vi "XYZStage.vi"() -> ()   [LabVIEW 2016]
uses:
  controls/Enum.ctl
  <vilib>/rvi/errors/niLvFpgaAdjustHostInterfaceError.vi
  <vilib>/rvi/interface/nirviReadWriteControl/nirviReadWriteControl.xnode
  controls/FPGAVIreferenceTypeDefScanEngine.ctl
  FPGA Bitfiles/lbniAFMControlle_scanControl_controllerFPGAPX_N4i+37z1gG8.lvbitx
  Course Project/support/Message Queue/Message Queue.lvlib
  NiFpgaLv.dll
panel:
  in  "x N (Discrete)":i32
  in  "Z axis":cluster{"Amplitude":dbl, "Frequency (Hz)":dbl}={"Amplitude"=0.1, "Frequency (Hz)"=100.0} {"Frequency (Hz)" scale=1.0..5000.0; "Amplitude" scale=0.0..10.0}
  in  "Z":cluster{"+":bool, "-":bool}
  in  "ClockDivider":i16=40
  in  "Increment":i16=30
  in  "Target":i16=30
  out "Output Scale":fxp<+/-,16,16>=16390.0
  in  "Max x":i16=32767
  in  "Min x":i16=-32767
  in  "Steps in a ramp":i16=31380
  in  "Steps":i16=32767
  in  "Y axis":cluster{"Amplitude":dbl, "Frequency (Hz)":dbl}={"Amplitude"=0.1, "Frequency (Hz)"=100.0} {"Frequency (Hz)" scale=1.0..5000.0; "Amplitude" scale=0.0..10.0}
  in  "X axis":cluster{"Amplitude":dbl, "Frequency (Hz)":dbl}={"Amplitude"=0.1, "Frequency (Hz)"=100.0} {"Frequency (Hz)" scale=1.0..5000.0; "Amplitude" scale=0.0..10.0}
  in  "X":cluster{"+":bool, "-":bool, "Stop":bool}
  in  "Y":cluster{"+":bool, "-":bool}
  in  "lock XY":bool
  in  "continuous":bool
  # "Joystick"
  # "XY stage"
  # "Z stage"
  # "Continuous"
  # "Discrete"
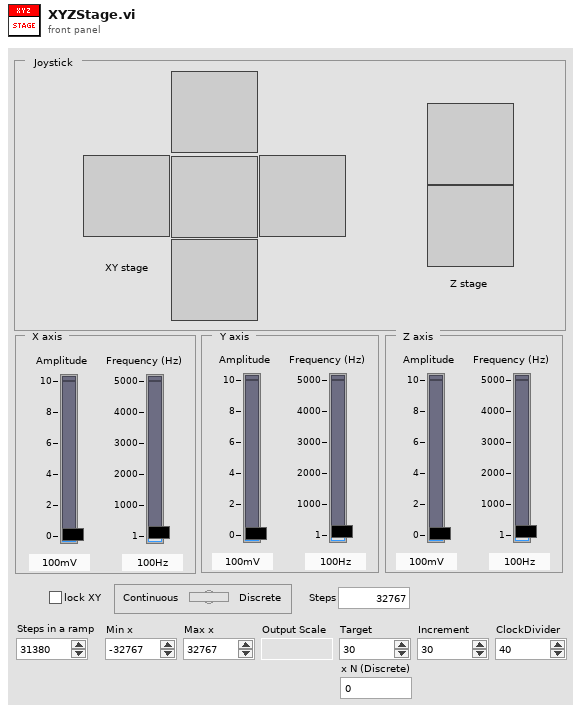
[diagram p1: front panel]
types:
  T1 = typedef "Message Queue.lvlib/All Message Queues.ctl" = cluster{"IU":refnum<queue>}
  T2 = typedef "Enum.ctl" = enum16{"Init", "Read", "Write"}
  T3 = typedef "FPGAVIreferenceTypeDefScanEngine.ctl" = refnum<k20>
  T4 = cluster{"InitialX":fxp<+/-,16,16>, "InitialY":fxp<+/-,16,16>, "InitialZ":fxp<+/-,16,16>}
  T5 = cluster{"target ":i16, "increment":i16, "ClockDivider":i16, "axis":enum16{"none", "x", "y", "z"}}
  T6 = cluster{"min_x":i16, "max_x":i16, "Total number of ramps":i16, "OutputScale":fxp<+/-,16,16>, "Steps in a ramp":i16}
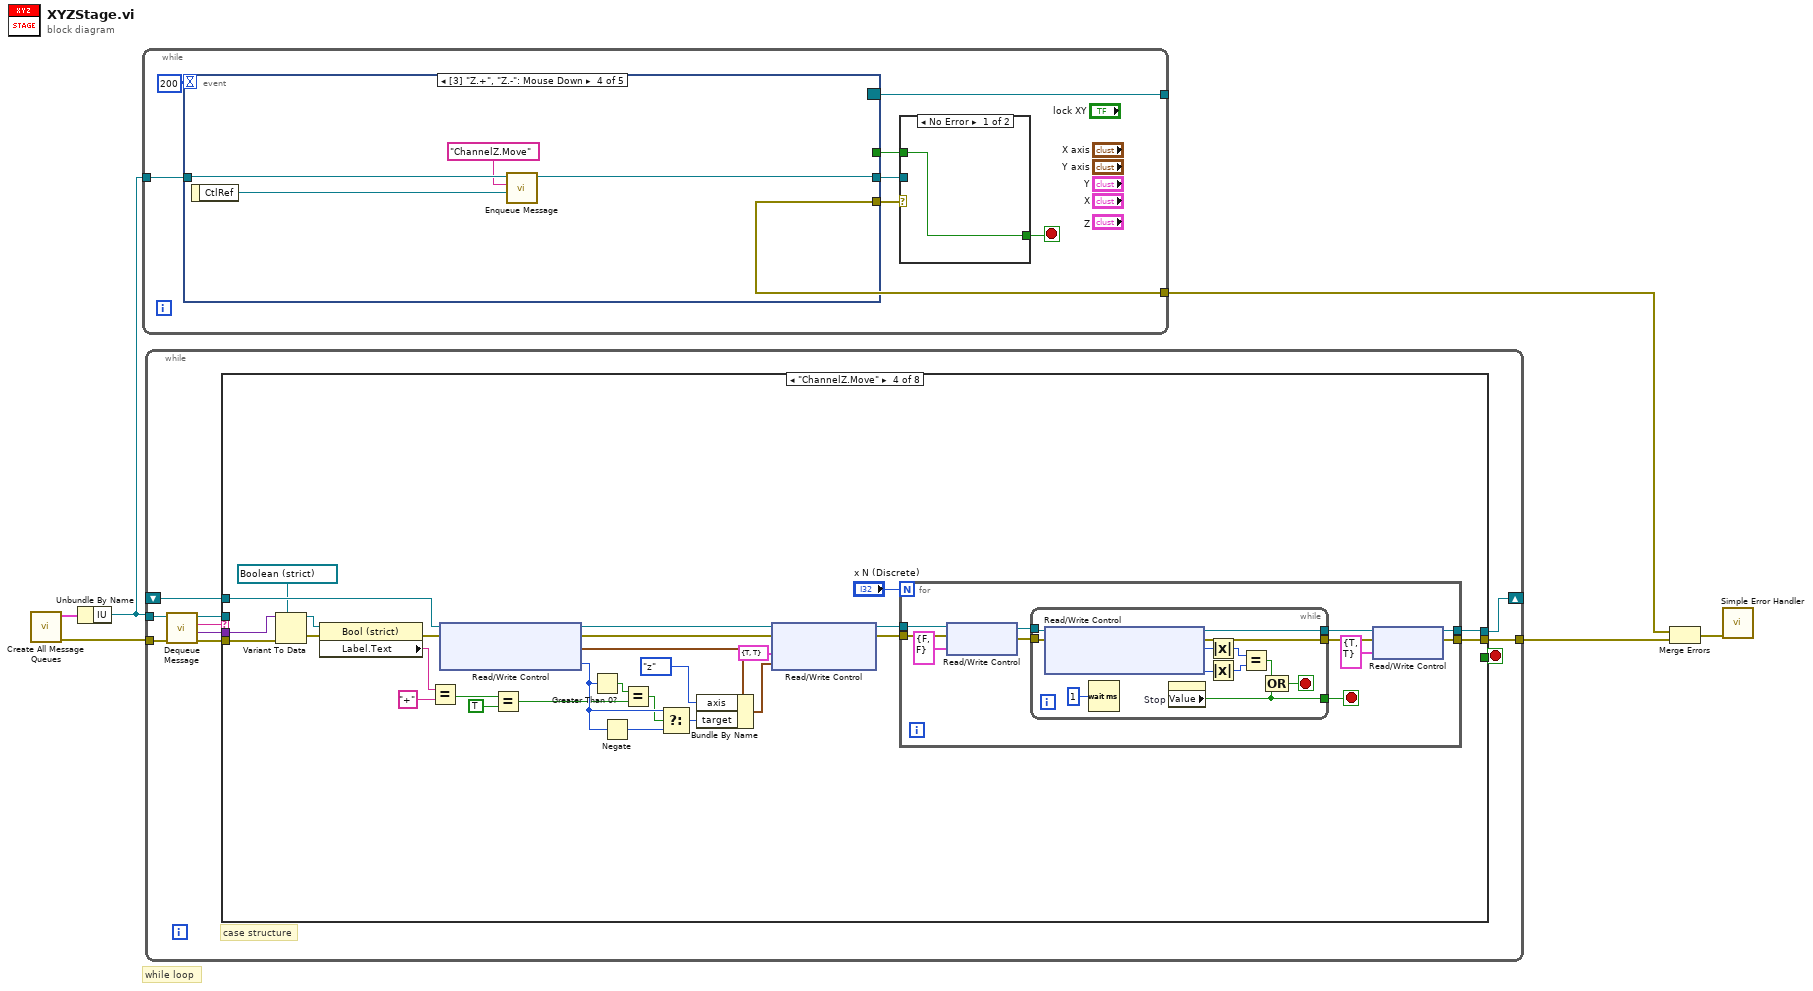
[diagram p0: block diagram]
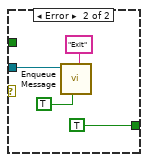
[diagram p2: hidden frame]
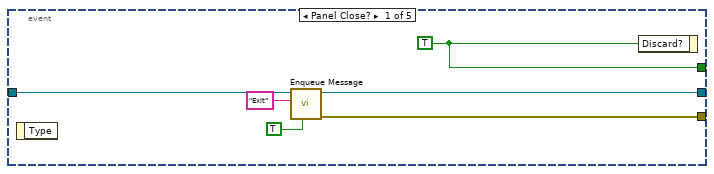
[diagram p3: hidden frame]
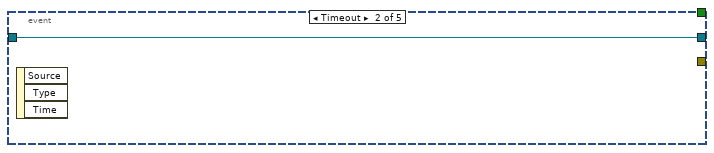
[diagram p4: hidden frame]
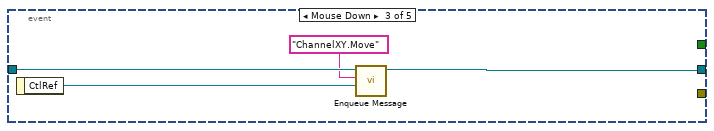
[diagram p5: hidden frame]
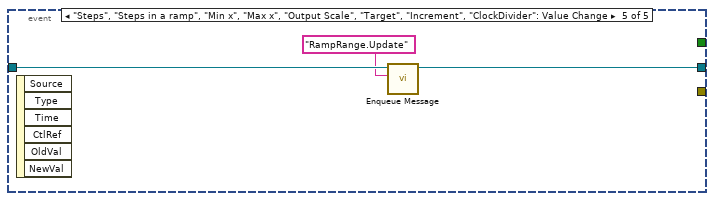
[diagram p6: hidden frame]
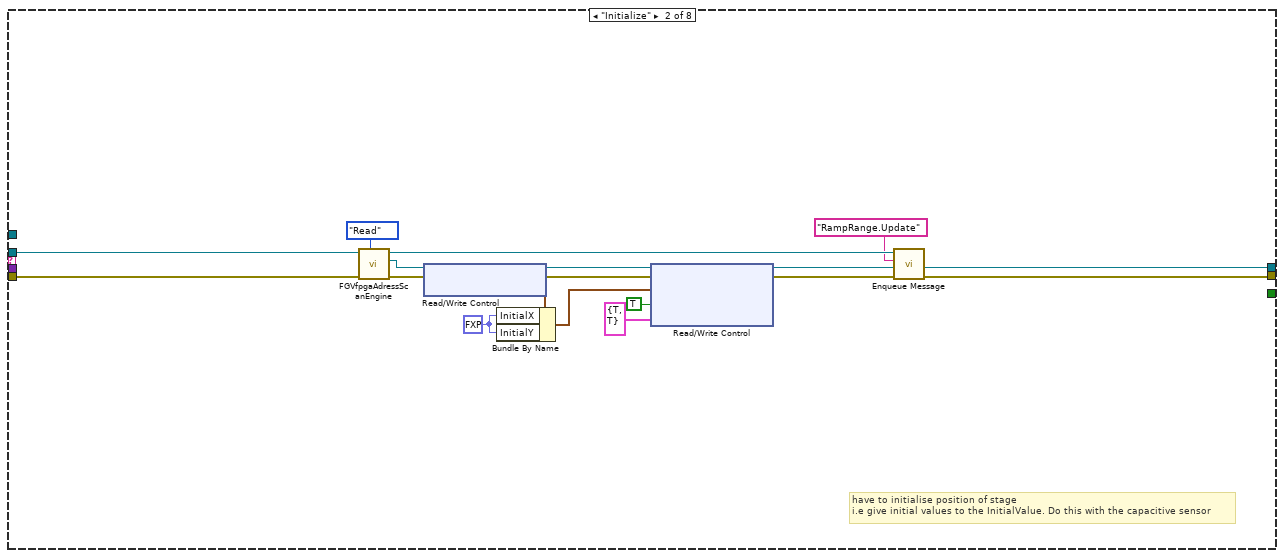
[diagram p8: hidden frame]
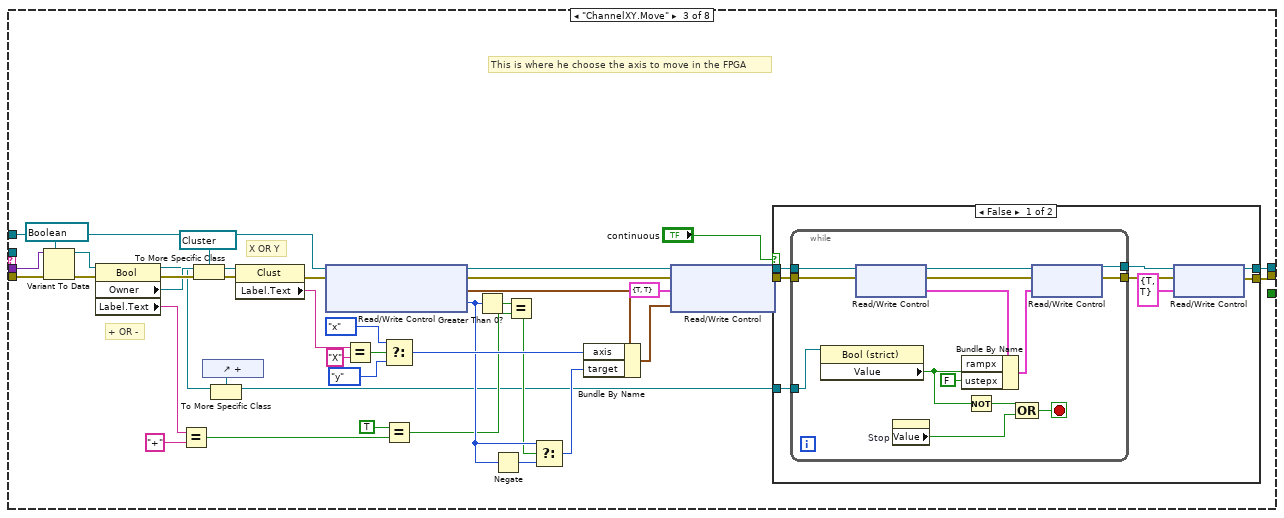
[diagram p9: hidden frame]
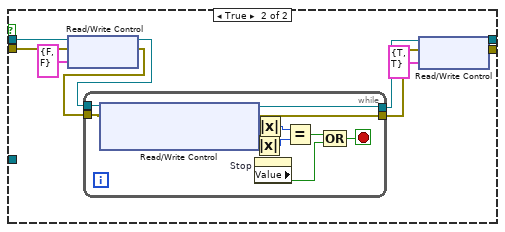
[diagram p10: hidden frame]
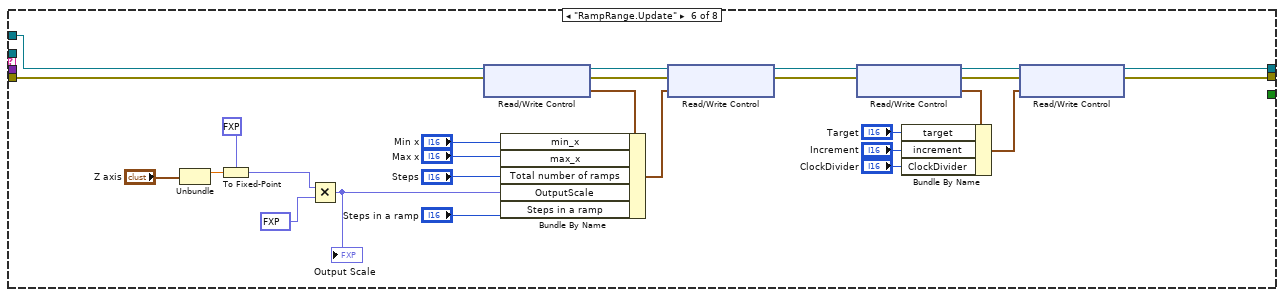
[diagram p12: hidden frame]
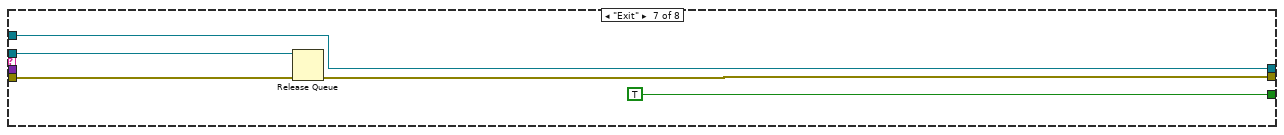
[diagram p13: hidden frame]
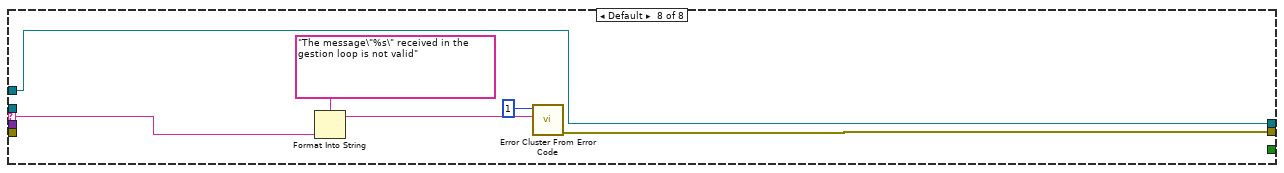
[diagram p14: hidden frame]
diagram:
  # "while loop"
  n1 = call "Create All Message Queues.vi"() -> ("ErrorOut"=w4:errorcluster, "MessageQueueOut"=w6:T1)  [unwired: 10 in]
  n2 = Unbundle By Name(w6) -> ("IU"=w5:refnum<queue>)
  n3 = while {
    tunnel: w5 -> [w13]
    tunnel: [w9] -> w1
    tunnel: [w8] -> _
    stop <- w11 stop-if-true
    n4 = event shown="[3] \"Z.+\", \"Z.-\": Mouse Down" {
      selector: _ -> [_ _ _ _ _]
      dyn-events: [_ _ _ _ _] -> w8
      timeout: 200 -> [_ _ _ _ _]
      tunnel: [w24 _ _ _ _] -> w12
      tunnel: w13 -> [w23 w25 w29 w33 w36]
      tunnel: [w22 _ _ _ _] -> w9
      tunnel: [w21 w25 w26 w31 w35] -> w10
      event Panel Close? {
        w24 = TRUE ("Rejeter ?")
        n5 = event-data() -> ()  [unwired: 1 in, 1 out]
        n6 = call "Enqueue Message.vi"("Prioritary message"=TRUE ("Message prioritaire ? (F)"), "Message"="Exit", "Queue"=w23) -> ("error out"=w22:errorcluster, "Queue dup."=w21:refnum<queue>)  [unwired: 7 in]
        n7 = event-data ("Event Filter Node")("Discard?"=w24) -> ()  [unwired: 1 in, 1 out]
      }
      event Timeout {
        n8 = event-data() -> ()  [unwired: 1 in, 3 out]
      }
      event "Y.+", "Y.-", "X.+", "X.-": Mouse Down {
        n9 = event-data() -> ("CtlRef"=w28:refnum<vi>)  [unwired: 1 in]
        n10 = call "Enqueue Message.vi"("Data"=w28, "Message"="ChannelXY.Move", "Queue"=w29) -> ("Queue dup."=w26:refnum<queue>)  [unwired: 7 in, 1 out]
      }
      event "Z.+", "Z.-": Mouse Down {
        n11 = event-data() -> ("CtlRef"=w30:refnum<vi>)  [unwired: 1 in]
        n12 = call "Enqueue Message.vi"("Data"=w30, "Message"="ChannelZ.Move", "Queue"=w33) -> ("Queue dup."=w31:refnum<queue>)  [unwired: 7 in, 1 out]
      }
      event "Steps", "Steps in a ramp", "Min x", "Max x", "Output Scale", "Target", "Increment", "ClockDivider", "Z axis.Amplitude": Value Change {
        n13 = event-data() -> ()  [unwired: 1 in, 6 out]
        n14 = call "Enqueue Message.vi"("Message"="RampRange.Update", "Queue"=w36) -> ("Queue dup."=w35:refnum<queue>)  [unwired: 8 in, 1 out]
      }
    }
    n15 = case shown="No Error" w9 {
      tunnel: [w14 TRUE ("Rejeter ?")] -> w11
      tunnel: w12 -> [w14 _]
      tunnel: w10 -> [_ w17]
      frame No Error {
      }
      frame Error {
        n16 = call "Enqueue Message.vi"("Prioritary message"=TRUE ("Message prioritaire ? (F)"), "Message"="Exit", "Queue"=w17) -> ()  [unwired: 7 in, 2 out]
      }
    }
  }
  n17 = while {
    tunnel: w5 -> [w40]
    tunnel: w4 -> [w44]
    tunnel: [w45] -> w2
    shift-right: [w38] -> _
    shift-left: _ -> [w37]
    stop <- w46 stop-if-true
    # "case structure"
    n18 = call "Dequeue Message.vi"("entrée d'erreur (pas d'erreur)"=w44, "File d'attente de messages"=w40) -> ("sortie d'erreur"=w43:errorcluster, "Données de message"=w42:variant, "Message"=w39:string, "File d'attente de message dup."=w41:refnum<queue>)  [unwired: 6 in]
    n19 = case "Conditions des messages" shown="\"ChannelZ.Move\"" w39 {
      selector: w39 -> [_ _ _ _ _ _ _ w237]
      tunnel: w41 -> [_ w64 _ _ _ _ w232 _]
      tunnel: w43 -> [w48 w62 w102 w154 w200 w226 w230 _]
      tunnel: [w48 w51 w65 w149 w200 w218 w229 w235] -> w45
      tunnel: [_ _ _ _ _ _ TRUE _] -> w46
      tunnel: w42 -> [_ _ w103 w155 _ _ _ _]
      tunnel: [w47 w54 w66 w150 w199 w219 w228 w233] -> w38
      tunnel: w37 -> [w47 _ w84 w156 w199 w208 w228 w233]
      frame "--------- Initialization ---------" {
      }
      frame "Initialize" {
        w56 = fxp<+/-,16,16> 0.0 ("InitialX")
        # "have to initialise position of stage\ni.e give initial values to the InitialValue. Do this with the capacitive sensor"
        n20 = call "FGVfpgaAdressScanEngine.vi"("Enum"=Enum."Read", "error in"=w62) -> ("error out"=w60:errorcluster, "FPGA.SEout"=w61:T3)  [unwired: 5 in, 3 out]
        n21 = xnode ("Read/Write Control")("FPGA VI Reference In"=w61, "error in"=w60) -> ("FPGA VI Reference Out"=w59:T3, "error out"=w58:errorcluster, "wfm.initialPositions"=w57:T4)
        n22 = Bundle By Name(cluster=w57, "InitialX"=w56, "InitialY"=w56) -> (w55:T4)
        n23 = xnode ("Read/Write Control")("FPGA VI Reference In"=w59, "error in"=w58, "wfm.initialPositions"=w55, "aio.wfm.enable"=TRUE, "wfm.reset"=cluster{"rampx":bool, "ustepx":bool} {"rampx"=TRUE, "ustepx"=TRUE} ("Reset")) -> ("FPGA VI Reference Out"=w54:T3, "error out"=w52:errorcluster)
        n24 = call "Enqueue Message.vi"("error in"=w52, "Message"="RampRange.Update", "Queue"=w64) -> ("error out"=w51:errorcluster)  [unwired: 7 in, 1 out]
      }
      frame "ChannelXY.Move" {
        # "This is where he choose the axis to move in the FPGA"
        # "+ OR -"
        # "X OR Y"
        n25 = Variant To Data(error in=w102, type=refnum<vi> refnum ("CtlRef"), Variant=w103) -> (data=w100:refnum<vi>, error out=w99:errorcluster)
        n26 = property class="Bool"(reference=w100, error in=w99) -> (reference out=w83:refnum<vi>, error out=w104:errorcluster, "Owner"=w98:refnum<vi>, "Label.Text"=w80:string)
        n27 = Equal?(x=w80, y="+") -> (x = y?=w73:bool)
        n28 = To More Specific Class(target class=refnum<vi> refnum ("Y"), reference=w98, error in=w104) -> (specific class reference=w96:refnum<vi>, error out=w95:errorcluster)
        n29 = control-ref of="+"() -> (w82:refnum<vi>)
        n30 = To More Specific Class(target class=w82, reference=w83) -> (specific class reference=w67:refnum<vi>)  [unwired: 1 in, 1 out]
        n31 = property class="Clust"(reference=w96, error in=w95) -> (error out=w94:errorcluster, "Label.Text"=w90:string)  [unwired: 1 out]
        n32 = xnode "Read/Write Control"("FPGA VI Reference In"=w84) -> ("FPGA VI Reference Out"=w93:T3, "wfm.Parameters"=w92:T5, "wfm.Parameters.target"=w76:i16)  [unwired: 1 in, 1 out]
        n33 = Equal?(x=w90, y="X") -> (x = y?=w88:bool)
        n34 = Select(t=enum16{"none", "x", "y", "z"}."x" ("axis"), s=w88, f=enum16{"none", "x", "y", "z"}."y" ("axis")) -> (s? t:f=w85:enum16{"none", "x", "y", "z"})
        n35 = Equal?(x=TRUE, y=w73) -> (x = y?=w72:bool)
        n36 = Greater Than 0?(x=w76) -> (x > 0?=w75:bool)
        n37 = Negate(x=w76) -> (-x=w77:i16)
        n38 = Equal?(x=w75, y=w72) -> (x = y?=w71:bool)
        n39 = Select(t=w76, s=w71, f=w77) -> (s? t:f=w78:i16)
        n40 = Bundle By Name(cluster=w92, "axis"=w85, "target"=w78) -> (w91:T5)
        n41 = xnode "Read/Write Control"("FPGA VI Reference In"=w93, "error in"=w94, "wfm.reset"=cluster{"rampx":bool, "ustepx":bool} {"rampx"=TRUE, "ustepx"=TRUE} ("Reset"), "wfm.Parameters"=w91) -> ("FPGA VI Reference Out"=w69:T3, "error out"=w68:errorcluster)
        n42 = case shown="False" "continuous" {
          tunnel: w69 -> [w112 w129]
          tunnel: w68 -> [w111 w128]
          tunnel: [w106 w130] -> w65
          tunnel: [w107 w131] -> w66
          tunnel: w67 -> [w105 _]
          frame False {
            n43 = while {
              tunnel: w112 -> [w123]
              tunnel: w111 -> [w122]
              tunnel: [w121] -> w109
              tunnel: [w120] -> w108
              tunnel: w105 -> [w117]
              stop <- w114 stop-if-true
              n44 = property class="Bool (strict)"(reference=w117) -> ("Value"=w116:bool)  [unwired: 1 in, 2 out]
              n45 = xnode "Read/Write Control"("FPGA VI Reference In"=w123, "error in"=w122) -> ("FPGA VI Reference Out"=w126:T3, "error out"=w125:errorcluster, "wfm.reset"=w119:cluster{"rampx":bool, "ustepx":bool})
              n46 = property on="Stop" class="Bool (strict)"() -> ("Value"=w113:bool)  [unwired: 2 in, 2 out]
              n47 = Bundle By Name(cluster=w119, "rampx"=w116, "ustepx"=FALSE) -> (w124:cluster{"rampx":bool, "ustepx":bool})
              n48 = Not(x=w116) -> (.not. x?=w115:bool)
              n49 = Compound Arithmetic op=OR(w115, w113) -> (w114:bool)
              n50 = xnode "Read/Write Control"("FPGA VI Reference In"=w126, "error in"=w125, "wfm.reset"=w124) -> ("FPGA VI Reference Out"=w121:T3, "error out"=w120:errorcluster)
            }
            n51 = xnode "Read/Write Control"("FPGA VI Reference In"=w109, "error in"=w108, "wfm.reset"=cluster{"rampx":bool, "ustepx":bool} {"rampx"=TRUE, "ustepx"=TRUE} ("Reset")) -> ("FPGA VI Reference Out"=w107:T3, "error out"=w106:errorcluster)
          }
          frame True {
            n52 = xnode "Read/Write Control"("FPGA VI Reference In"=w129, "error in"=w128, "wfm.reset"=cluster{"rampx":bool, "ustepx":bool} {"rampx"=FALSE, "ustepx"=FALSE}) -> ("FPGA VI Reference Out"=w136:T3, "error out"=w135:errorcluster)
            n53 = while {
              tunnel: w136 -> [w142]
              tunnel: w135 -> [w143]
              tunnel: [w141] -> w133
              tunnel: [w140] -> w132
              stop <- w139 stop-if-true
              n54 = xnode "Read/Write Control"("FPGA VI Reference In"=w142, "error in"=w143) -> ("FPGA VI Reference Out"=w141:T3, "error out"=w140:errorcluster, "wfm.Parameters.target"=w147:i16, "wfm.rampIndex.NextRamp"=w145:i16)
              n55 = Absolute Value(x=w145) -> (abs(x)=w144:i16)
              n56 = Absolute Value(x=w147) -> (abs(x)=w146:i16)
              n57 = property on="Stop" class="Bool (strict)"() -> ("Value"=w137:bool)  [unwired: 2 in, 2 out]
              n58 = Equal?(x=w146, y=w144) -> (x = y?=w138:bool)
              n59 = Compound Arithmetic op=OR(w138, w137) -> (w139:bool)
            }
            n60 = xnode "Read/Write Control"("FPGA VI Reference In"=w133, "error in"=w132, "wfm.reset"=cluster{"rampx":bool, "ustepx":bool} {"rampx"=TRUE, "ustepx"=TRUE} ("Reset")) -> ("FPGA VI Reference Out"=w131:T3, "error out"=w130:errorcluster)
          }
        }
      }
      frame "ChannelZ.Move" {
        n61 = Variant To Data(error in=w154, type=refnum<vi> refnum ("reference"), Variant=w155) -> (data=w152:refnum<vi>, error out=w151:errorcluster)
        n62 = property class="Bool (strict)"(reference=w152, error in=w151) -> (error out=w165:errorcluster, "Label.Text"=w164:string)  [unwired: 1 out]
        n63 = Equal?(x=w164, y="+" ("x")) -> (x = y?=w168:bool)
        n64 = xnode "Read/Write Control"("FPGA VI Reference In"=w156, "error in"=w165) -> ("FPGA VI Reference Out"=w172:T3, "error out"=w173:errorcluster, "wfm.Parameters"=w166:T5, "wfm.Parameters.target"=w167:i16)
        n65 = Equal?(x=w168, y=TRUE) -> (x = y?=w160:bool)
        n66 = Greater Than 0?(x=w167) -> (x > 0?=w161:bool)
        n67 = Negate(x=w167) -> (-x=w157:i16)
        n68 = Equal?(x=w161, y=w160) -> (x = y?=w158:bool)
        n69 = Select(t=w167, s=w158, f=w157) -> (s? t:f=w159:i16)
        n70 = Bundle By Name(cluster=w166, "axis"=enum16{"none", "x", "y", "z"}."z", "target"=w159) -> (w171:T5)
        n71 = xnode "Read/Write Control"("FPGA VI Reference In"=w172, "error in"=w173, "wfm.reset"=cluster{"rampx":bool, "ustepx":bool} {"rampx"=TRUE, "ustepx"=TRUE} ("Reset"), "wfm.Parameters"=w171) -> ("FPGA VI Reference Out"=w174:T3, "error out"=w175:errorcluster)
        n72 = for {
          N: "x N (Discrete)" -> [_]
          tunnel: w174 -> [w179]
          tunnel: [w178] -> w150
          tunnel: w175 -> [w180]
          tunnel: [w177] -> w149
          stop <- w176 stop-if-true
          n73 = xnode "Read/Write Control"("FPGA VI Reference In"=w179, "error in"=w180, "wfm.reset"=cluster{"rampx":bool, "ustepx":bool} {"rampx"=FALSE, "ustepx"=FALSE} ("Reset")) -> ("FPGA VI Reference Out"=w185:T3, "error out"=w184:errorcluster)
          n74 = while {
            tunnel: w185 -> [w192]
            tunnel: w184 -> [w191]
            tunnel: [w190] -> w183
            tunnel: [w189] -> w182
            tunnel: [w187] -> w176
            stop <- w193 stop-if-true
            n75 = xnode "Read/Write Control"("FPGA VI Reference In"=w192, "error in"=w191) -> ("FPGA VI Reference Out"=w189:T3, "error out"=w190:errorcluster, "wfm.Parameters.target"=w194:i16, "wfm.rampIndex.NextRamp"=w195:i16)
            n76 = Wait (ms)(milliseconds to wait=u32 1) -> ()  [unwired: 1 out]
            n77 = property on="Stop" class="Bool (strict)"() -> ("Value"=w187:bool)  [unwired: 2 in, 2 out]
            n78 = Absolute Value(x=w194) -> (abs(x)=w196:i16)
            n79 = Absolute Value(x=w195) -> (abs(x)=w197:i16)
            n80 = Equal?(x=w196, y=w197) -> (x = y?=w198:bool)
            n81 = Compound Arithmetic op=OR(w198, w187) -> (w193:bool)
          }
          n82 = xnode "Read/Write Control"("FPGA VI Reference In"=w182, "error in"=w183, "wfm.reset"=cluster{"rampx":bool, "ustepx":bool} {"rampx"=TRUE, "ustepx"=TRUE} ("Reset")) -> ("FPGA VI Reference Out"=w178:T3, "error out"=w177:errorcluster)
        }
      }
      frame "Joystick.Pressed" {
      }
      frame "RampRange.Update" {
        n83 = Unbundle("Z axis") -> ("Amplitude"=w202:dbl)  [unwired: 1 out]
        n84 = To Fixed-Point(fixed-point type=fxp<+/-,16,16> 0.0, number=w202) -> (fixed-point=w203:fxp<+/-,16,16>)
        n85 = Multiply(x=w203, y=fxp<+/-,16,16> 1780.0) -> (x*y=w204:fxp<+/-,16,16>)
        "Output Scale" <- w204
        n86 = xnode "Read/Write Control"("FPGA VI Reference In"=w208, "error in"=w226) -> ("FPGA VI Reference Out"=w207:T3, "error out"=w227:errorcluster, "wfm.rampRange"=w225:T6)
        n87 = Bundle By Name(cluster=w225, "min_x"="Min x", "max_x"="Max x", "Total number of ramps"="Steps", "OutputScale"=w204, "Steps in a ramp"="Steps in a ramp") -> (w224:T6)
        n88 = xnode "Read/Write Control"("FPGA VI Reference In"=w207, "error in"=w227, "wfm.rampRange"=w224) -> ("FPGA VI Reference Out"=w215:T3, "error out"=w214:errorcluster)
        n89 = xnode "Read/Write Control"("FPGA VI Reference In"=w215, "error in"=w214) -> ("FPGA VI Reference Out"=w217:T3, "error out"=w216:errorcluster, "wfm.Parameters"=w213:T5)
        n90 = Bundle By Name(cluster=w213, "target"="Target", "increment"="Increment", "ClockDivider"="ClockDivider") -> (w212:T5)
        n91 = xnode "Read/Write Control"("FPGA VI Reference In"=w217, "error in"=w216, "wfm.Parameters"=w212) -> ("FPGA VI Reference Out"=w219:T3, "error out"=w218:errorcluster)
      }
      frame "Exit" {
        n92 = Release Queue(queue=w232, error in (no error)=w230) -> (error out=w229:errorcluster)  [unwired: 1 in, 2 out]
      }
      frame Default {
        n93 = Format Into String(format string="The message\"%s\" received in the gestion loop is not valid" ("Texte de message d'erreur inconnu"), w237) -> (resulting string=w234:string)  [unwired: 2 in, 1 out]
        n94 = call <vilib>:"Error Cluster From Error Code.vi"("error message (\"\")"=w234, "error code (0)"=1 ("code d'erreur (0)")) -> ("error out"=w235:errorcluster)  [unwired: 7 in]
      }
    }
  }
  n95 = Merge Errors(w1, w2) -> (w3:errorcluster)
  n96 = call <vilib>:"Simple Error Handler.vi"("error in (no error)"=w3) -> ()  [unwired: 4 in, 5 out]
